vi "Read.vi"(8 "error in (no error)":errorcluster, 9 "bytes to read":i32, 11 "pipe reader in":refnum<data-value>) -> (0 "error out":errorcluster, 1 "bytes read":i32, 2 "data":string, 3 "pipe reader out":refnum<data-value>)   [LabVIEW 2013, in "Pipes.lvlib" / "Unix Pipe Reader.lvclass"]
doc: "This VI reads a certain number of bytes from the provided pipe endpoint."
uses:
  Unix Pipe Reader.lvclass
  Unix Pipe/Unix Pipe.lvclass/Unix Pipe.ctl
  Unix Pipe/Unix Pipe.lvclass
  Pipes.lvlib
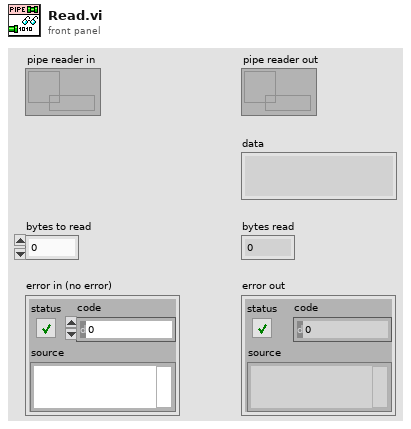
[diagram p1: front panel]
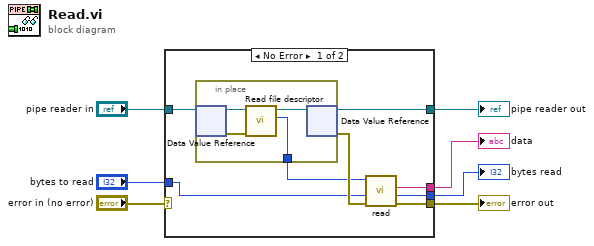
[diagram p0: block diagram]
diagram:
  n1 = case shown="No Error" "error in (no error)" {
    selector: "error in (no error)" -> [_ w20]
    tunnel: "pipe reader in" -> [w14 w21]
    tunnel: [w13 w21] -> w5
    tunnel: "bytes to read" -> [w12 _]
    tunnel: [w10 w20] -> w3
    tunnel: [w9 _] -> w2
    tunnel: [w8 _] -> w1
    frame No Error {
      n2 = in-place {
        in-place-border: [w17] -> w11
        n3 = in-place-dvr #1(w14) -> (w19:refnum<class "Unix Pipe Reader.lvclass">, w18:errorcluster)
        n4 = call "Read file descriptor.vi"("error in (no error)"=w18, "Unix Pipe in"=w19) -> ("file descriptor"=w17:i32, "Unix Pipe out"=w16:refnum<class "Unix Pipe Reader.lvclass">)  [unwired: 7 in, 1 out]
        n5 = in-place-dvr #1(w16) -> (w13:refnum<data-value>, w15:errorcluster)
      }
      n6 = call "read.vi"("error in (no error)"=w15, "bytes to read"=w12, "file descriptor in"=w11) -> ("error out"=w10:errorcluster, "bytes read"=w9:i32, "data"=w8:string)  [unwired: 5 in, 1 out]
    }
    frame Error {
    }
  }
  "error out" <- w3
  "pipe reader out" <- w5
  "bytes read" <- w2
  "data" <- w1
